vi "Fire User Event - ExitAllLoops.vi"(8 "error in (no error)":errorcluster, 10 "user event ExitEventLoop":refnum<user-event>) -> (0 "error out":errorcluster)   [LabVIEW 2018, in "UserEvent-ExitEventLoop.lvlib"]
doc: "Send the Stop event to stop the Event Handling Loop.\n\nBolder Software LLC"
uses:
  UserEvent-ExitEventLoop.lvlib
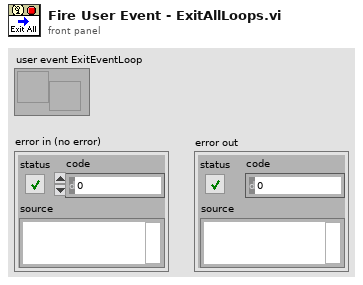
[diagram p1: front panel]
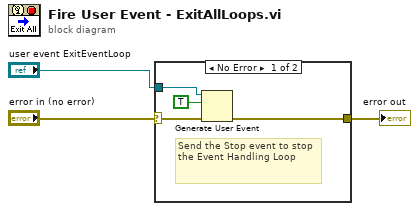
[diagram p0: block diagram]
diagram:
  n1 = case shown="No Error" "error in (no error)" {
    selector: "error in (no error)" -> [w4 w8]
    tunnel: [w6 w8] -> w1
    tunnel: "user event ExitEventLoop" -> [w5 _]
    frame No Error {
      # "Send the Stop event to stop the Event Handling Loop"
      n2 = Generate User Event(user event=w5, event data cluster=TRUE ("event data"), error in=w4) -> (error out=w6:errorcluster)  [unwired: 1 in, 1 out]
    }
    frame Error {
    }
  }
  "error out" <- w1
